vi "GlobalVars.vi"() -> ()   [LabVIEW 2014]
panel:
  in  "Motor Movement Completed":bool
  in  "Motor Movement Commant Sent":bool
  out "GoMove Notifier":refnum<notifier>
  in  "Motor Reset":bool=TRUE
  out "MovementSignal":dbl[](array[numeric])
  out "AODPositionUpdateTime":dbl
  out "MovementDetectionTime":dbl
  out "VolumeData":i32[][](array[numeric])
  out "MotionAnalysis":refnum<queue>
  in  "Scanning":bool
  in  "Sampling Interval (sec)":dbl
  in  "Number of Scan Planes":i32
  in  "VI Open":bool
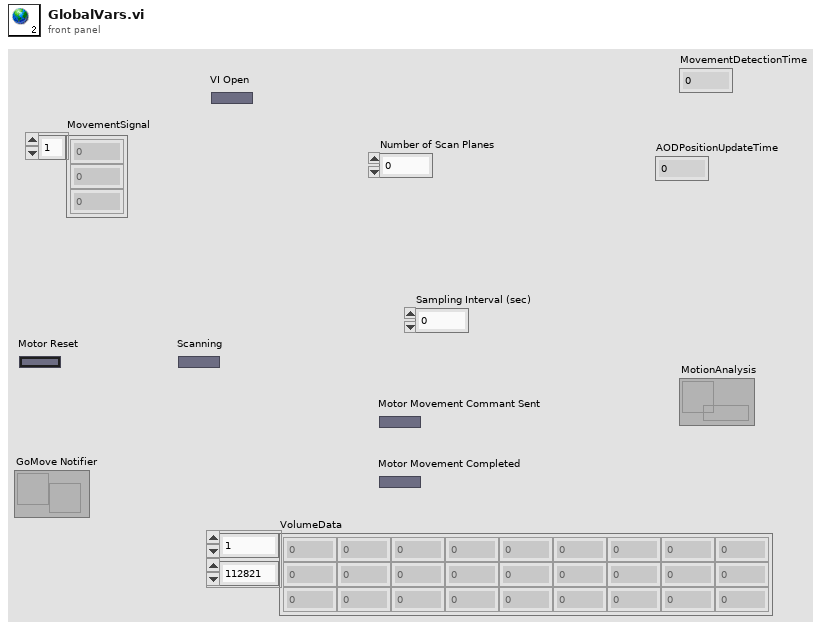
[diagram p1: front panel]
diagram:
